vi "change_experimentController.vi"(8 "error in (no error)":errorcluster, 10 "experimentControllers":T1[](array[typedef]), 11 "control references in":T2) -> (0 "error out":errorcluster)   [LabVIEW 2010]
uses:
  type_definitions/clusters/controls_refs.ctl
  common/clusters/plugin_specification.ctl
  components/ExperimentController/GenericExperimentController/GenericExperimentController/GenericExperimentController.lvclass
  common/classes/ErrorController/ErrorController/class_data.vi
  common/classes/GenericComponent/GenericComponent/GenericComponent.lvclass
  common/classes/ErrorController/ErrorController/ErrorController.lvclass
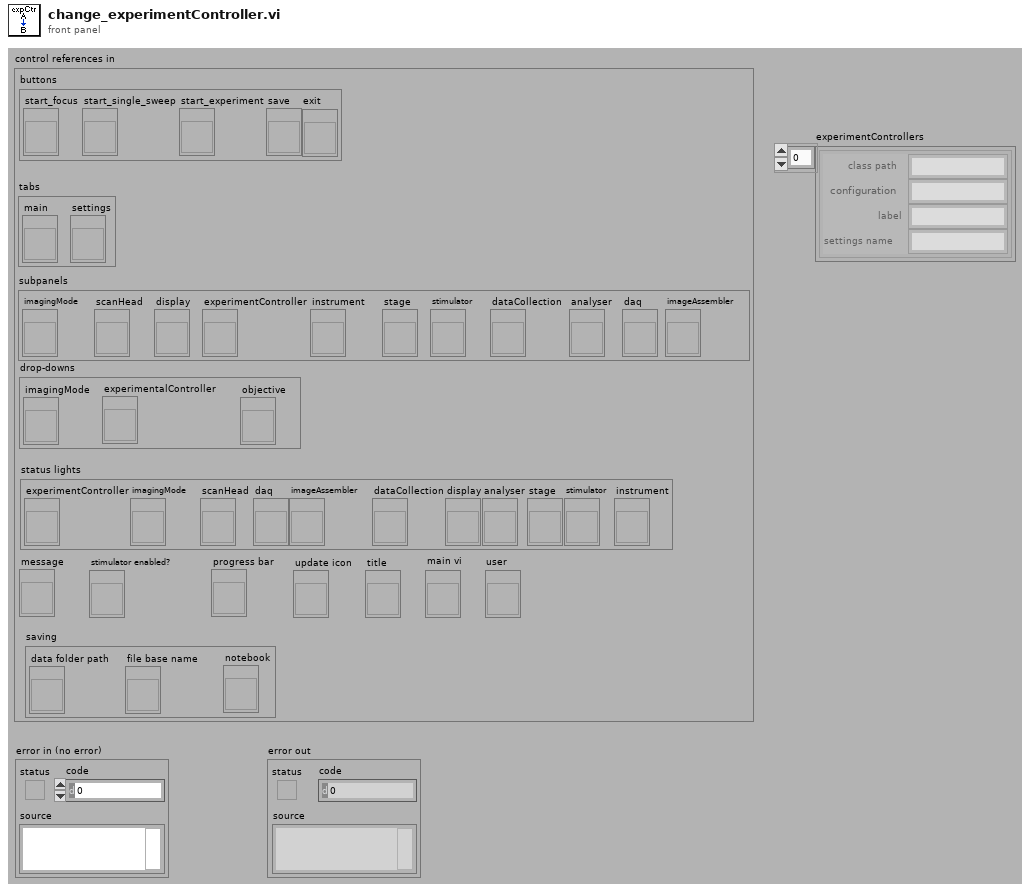
[diagram p1: front panel]
types:
  T1 = typedef "plugin_specification.ctl" = cluster{"class path":string, "configuration":string, "label":string, "settings name":string}
  T2 = typedef "controls_refs.ctl" = cluster{"buttons":cluster{"start_focus":refnum<vi>, "start_single_sweep":refnum<vi>, "start_experiment":refnum<vi>, "save":refnum<vi>, "exit":refnum<vi>}, "tabs":cluster{"main":refnum<vi>, "settings":refnum<vi>}, "subpanels":cluster{"imagingMode":refnum<vi>, "scanHead":refnum<vi>, "display":refnum<vi>, "experimentController":refnum<vi>, "instrument":refnum<vi>, "stage":refnum<vi>, "stimulator":refnum<vi>, "dataCollection":refnum<vi>, "analyser":refnum<vi>, "daq":refnum<vi>, "imageAssembler":refnum<vi>}, "drop-downs":cluster{"imagingMode":refnum<vi>, "experimentalController":refnum<vi>, "objective":refnum<vi>}, "status lights":cluster{"experimentController":refnum<vi>, "imagingMode":refnum<vi>, "scanHead":refnum<vi>, "daq":refnum<vi>, "imageAssembler":refnum<vi>, "dataCollection":refnum<vi>, "display":refnum<vi>, "analyser":refnum<vi>, "stage":refnum<vi>, "stimulator":refnum<vi>, "instrument":refnum<vi>}, "message":refnum<vi>, "stimulator enabled?":refnum<vi>, "saving":cluster{"data folder path":refnum<vi>, "file base name":refnum<vi>, "notebook":refnum<vi>}, "progress bar":refnum<vi>, "update icon":refnum<vi>, "title":refnum<vi>, "main vi":refnum<vi>, "user":refnum<vi>}
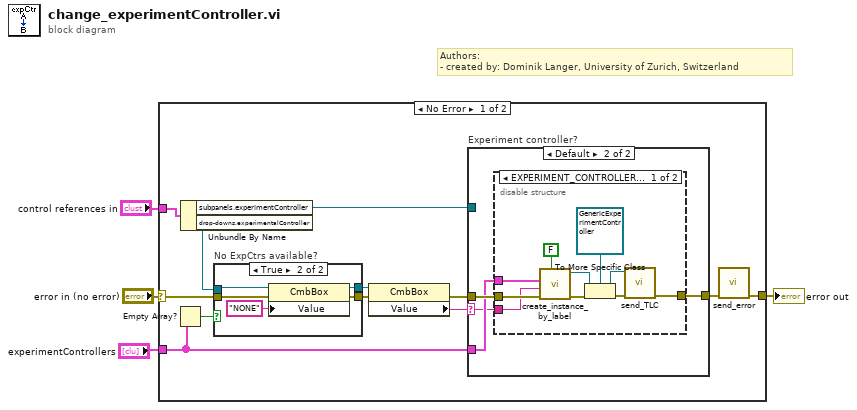
[diagram p0: block diagram]
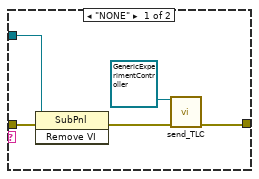
[diagram p3: hidden frame]
diagram:
  # "Authors: \n- created by: Dominik Langer, University of Zurich, Switzerland"
  n1 = case shown="No Error" "error in (no error)" {
    selector: "error in (no error)" -> [w11 w44]
    tunnel: "control references in" -> [w16 _]
    tunnel: [w6 w44] -> w3
    tunnel: "experimentControllers" -> [w12 _]
    frame No Error {
      n2 = Empty Array?(array=w12) -> (empty?=w7:bool)
      n3 = Unbundle By Name(w16) -> ("subpanels.experimentController"=w13:refnum<vi>, "drop-downs.experimentalController"=w9:refnum<vi>)
      n4 = case "No ExpCtrs available?" shown="True" w7 {
        tunnel: w11 -> [w17 w23]
        tunnel: [w17 w22] -> w10
        tunnel: w9 -> [w18 w20]
        tunnel: [w18 w19] -> w8
        frame False {
        }
        frame True {
          n5 = property class="CmbBox"(reference=w20, error in=w23, "Value"="NONE") -> (reference out=w19:refnum<vi>, error out=w22:errorcluster)
        }
      }
      n6 = property class="CmbBox"(reference=w8, error in=w10) -> (error out=w15:errorcluster, "Value"=w14:string)  [unwired: 1 out]
      n7 = case "Experiment controller?" shown="Default" w14 {
        selector: w14 -> [_ w29]
        tunnel: w15 -> [w28 w32]
        tunnel: w12 -> [_ w31]
        tunnel: [w26 w30] -> w5
        tunnel: w13 -> [w24 _]
        frame "NONE" {
          n8 = invoke on="Invoke Node" class="SubPnl" method="Remove VI"(reference=w24, error in=w28) -> (error out=w27:errorcluster)  [unwired: 1 in, 2 out]
          n9 = call-dynamic "send_TLC.vi"("error in (no error)"=w27, "GenericToplevelComponent in"=refnum<class "GenericExperimentController.lvclass"> refnum ("GenericExperimentController.lvclass")) -> ("error out"=w26:errorcluster)  [unwired: 9 out]
        }
        frame Default {
          n10 = disable-structure shown="EXPERIMENT_CONTROLLER==1" {
            disable-tunnel: w32 -> [w38 w43]
            disable-tunnel: w31 -> [w36 _]
            disable-tunnel: [w41 w43] -> w30
            disable-tunnel: w29 -> [w35 _]
            frame condition #0 (active) {
              n11 = call "create_instance_by_label.vi"("call constructor?"=FALSE, "error in (no error)"=w38, "label"=w35, "configuration list"=w36) -> ("error out"=w37:errorcluster, "GenericPlugin out"=w34:refnum<class "GenericComponent.lvclass">)  [unwired: 6 out]
              n12 = To More Specific Class(target class=refnum<class "GenericExperimentController.lvclass"> refnum ("GenericExperimentController.lvclass"), reference=w34, error in=w37) -> (specific class reference=w39:refnum<class "GenericExperimentController.lvclass">, error out=w40:errorcluster)
              n13 = call-dynamic "send_TLC.vi"("error in (no error)"=w40, "GenericToplevelComponent in"=w39) -> ("error out"=w41:errorcluster)  [unwired: 9 out]
            }
            frame condition #1 {
            }
          }
        }
      }
      n14 = call "send_error.vi"("error in (no error)"=w5) -> ("error out"=w6:errorcluster)  [unwired: 10 in]
    }
    frame Error {
    }
  }
  "error out" <- w3
